vi "FeedbackDecode_20200902.vi"() -> ()   [LabVIEW 2016] (continued)
                n1304 = call "FeedbackDecode_WriteTextEOL.vi"("text"=w1184, "refnum in"=w1190) -> ()  [unwired: 8 in, 2 out]
                n1305 = Initialize Array(0.0 ("element"), 2 ("dimension size"), 12 ("dimension size")) -> (w1179:dbl[][])
                n1306 = Bundle By Name(cluster=w1191, "EventStr"=w1184, "TrialCnt"=w1179) -> (w1183:T5)
                n1307 = local read "LoopCnt"() -> (w1193:u64)
                n1308 = local write "ResetCorr"(TRUE ("ResetCorr")) -> ()
                n1309 = call "FeedbackDecode_MLComCtrl.vi"("DecodeClustIn"=w1183, "Mode"=T19."SendEvent") -> ("DecodeClustOut"=w1178:T5)  [unwired: 6 in, 3 out]
                n1310 = local write "BaseCnt1"(w1193) -> ()
                n1311 = local write "DecodeClust"(w1178) -> ()
              }
            }
          }
          event Value Change {
            n1312 = event-data() -> ("CtlRef"=w1205:refnum<vi>)  [unwired: 1 in, 5 out]
            n1313 = property class="Ctl"(reference=w1205) -> ("Label.Text"=w1204:string)  [unwired: 1 in, 2 out]
            n1314 = case shown="\"ResetTrial\"" w1204 {
              frame "", Default {
              }
              frame "ResetTrial" {
                n1315 = local read "State"() -> (w1207:T16)
                n1316 = case shown="\"Acquire Start\", Default" w1207 {
                  frame "Initialize" {
                    n1317 = local read "DecodeClust"() -> (w1210:T5)
                    n1318 = Bundle By Name(cluster=w1210, "CtrlButtons.ResetTrial"=FALSE) -> (w1209:T5)
                    n1319 = local write "DecodeClust"(w1209) -> ()
                  }
                  frame "Acquire Start", Default {
                    n1320 = local read "NIPTime"() -> (w1215:dbl)
                    n1321 = local read "LoopCnt"() -> (w1219:u64)
                    n1322 = call-poly "FeedbackDecode_VariablesToString.vi"("Format"="%0.0f", "ValueIn"=w1215, "FieldName"="NIPTime" ("Key Word")) -> ("StringOut"=w1212:string)  [unwired: 4 in]
                    n1323 = Format Into String(w1219) -> (resulting string=w1211:string)  [unwired: 3 in, 1 out]
                    n1324 = local read "EventParamsFID"() -> (w1223:refnum<file>)
                    n1325 = local read "DecodeClust"() -> (w1224:T5)
                    n1326 = Concatenate Strings("ResetTrial:SS.EventID=" ("string"), w1211) -> (w1218:string)
                    n1327 = Concatenate Strings(w1218, ";", w1212) -> (w1217:string)
                    n1328 = call "FeedbackDecode_WriteTextEOL.vi"("text"=w1217, "refnum in"=w1223) -> ()  [unwired: 8 in, 2 out]
                    n1329 = Bundle By Name(cluster=w1224, "EventStr"=w1217) -> (w1216:T5)
                    n1330 = call "FeedbackDecode_MLComCtrl.vi"("DecodeClustIn"=w1216, "Mode"=T19."SendEvent") -> ()  [unwired: 6 in, 4 out]
                  }
                }
              }
            }
            n1331 = local read "MvntBuilder"() -> (w1196:T6)
            n1332 = Unbundle By Name(w1196) -> ("Mode"=w1203:enum16{"Selected", "Block", "Random"}, "NTrials"=w1200:dbl, "MvntList"=w1199:T24)
            n1333 = property on="MvntList" class="Arr (strict)"() -> ("Index Values"=w1197:u32[])  [unwired: 2 in, 2 out]
            n1334 = Array Size(array=w1199) -> (size(s)=w1198:i32)
            n1335 = Index Array(array=w1197) -> (element=w1201:u32)  [unwired: 1 in]
            n1336 = call "FeedbackDecode_GenRandBlockIdxs2.vi"("Mode"=w1203, "Reset"=TRUE, "NumTrials"=w1200, "NumIdxs"=w1198, "CurrIdx"=w1201) -> ("Perc"=w1195:dbl)  [unwired: 1 out]
            n1337 = Bundle By Name(cluster=w1196, "PercTrials"=w1195) -> (w1194:T6)
            n1338 = local write "MvntBuilder"(w1194) -> ()
          }
          event Value Change {
            n1339 = event-data() -> ("NewVal"=w1225:bool)  [unwired: 1 in, 5 out]
            n1340 = case shown="True" w1225 {
              frame False {
                n1341 = local read "LoopCnt"() -> (w1237:u64)
                n1342 = local read "NIPTime"() -> (w1231:dbl)
                n1343 = Format Into String(w1237) -> (resulting string=w1227:string)  [unwired: 3 in, 1 out]
                n1344 = call-poly "FeedbackDecode_VariablesToString.vi"("Format"="%0.0f", "ValueIn"=w1231, "FieldName"="NIPTime" ("Key Word")) -> ("StringOut"=w1228:string)  [unwired: 4 in]
                n1345 = Concatenate Strings("DisableHideSpheres:SS.EventID=" ("string"), w1227) -> (w1236:string)
                n1346 = local read "EventParamsFID"() -> (w1234:refnum<file>)
                n1347 = local read "DecodeClust"() -> (w1240:T5)
                n1348 = Concatenate Strings(w1236, ";SS.HideSpheres=0;" ("EventStr"), w1228) -> (w1233:string)
                n1349 = call "FeedbackDecode_WriteTextEOL.vi"("text"=w1233, "refnum in"=w1234) -> ()  [unwired: 8 in, 2 out]
                n1350 = Bundle By Name(cluster=w1240, "EventStr"=w1233) -> (w1232:T5)
                n1351 = call "FeedbackDecode_MLComCtrl.vi"("DecodeClustIn"=w1232, "Mode"=T19."SendEvent") -> ()  [unwired: 6 in, 4 out]
              }
              frame True {
                n1352 = local read "LoopCnt"() -> (w1251:u64)
                n1353 = local read "NIPTime"() -> (w1245:dbl)
                n1354 = Format Into String(w1251) -> (resulting string=w1241:string)  [unwired: 3 in, 1 out]
                n1355 = Concatenate Strings("EnableHideSpheres:SS.EventID=" ("string"), w1241) -> (w1250:string)
                n1356 = call-poly "FeedbackDecode_VariablesToString.vi"("Format"="%0.0f", "ValueIn"=w1245, "FieldName"="NIPTime" ("Key Word")) -> ("StringOut"=w1242:string)  [unwired: 4 in]
                n1357 = local read "EventParamsFID"() -> (w1248:refnum<file>)
                n1358 = local read "DecodeClust"() -> (w1254:T5)
                n1359 = Concatenate Strings(w1250, ";SS.HideSpheres=1;" ("EventStr"), w1242) -> (w1247:string)
                n1360 = call "FeedbackDecode_WriteTextEOL.vi"("text"=w1247, "refnum in"=w1248) -> ()  [unwired: 8 in, 2 out]
                n1361 = Bundle By Name(cluster=w1254, "EventStr"=w1247) -> (w1246:T5)
                n1362 = call "FeedbackDecode_MLComCtrl.vi"("DecodeClustIn"=w1246, "Mode"=T19."SendEvent") -> ()  [unwired: 6 in, 4 out]
              }
            }
          }
          event Value Change {
            n1363 = event-data() -> ("NewVal"=w1256:T44)  [unwired: 1 in, 5 out]
            n1364 = Format Into String(w1256) -> (resulting string=w1255:string)  [unwired: 3 in, 1 out]
            n1365 = local read "LoopCnt"() -> (w1265:u64)
            n1366 = call-poly "FeedbackDecode_VariablesToString.vi"("ValueIn"=w1255, "FieldName"="KalmanType") -> ("StringOut"=w1272:string)  [unwired: 5 in]
            n1367 = local read "NIPTime"() -> (w1261:dbl)
            n1368 = Format Into String(w1265) -> (resulting string=w1257:string)  [unwired: 3 in, 1 out]
            n1369 = local read "EventParamsFID"() -> (w1269:refnum<file>)
            n1370 = local read "DecodeClust"() -> (w1270:T5)
            n1371 = Concatenate Strings("ChangeKalmanType:SS.EventID=" ("string"), w1257) -> (w1264:string)
            n1372 = call-poly "FeedbackDecode_VariablesToString.vi"("Format"="%0.0f", "ValueIn"=w1261, "FieldName"="NIPTime" ("Key Word")) -> ("StringOut"=w1258:string)  [unwired: 4 in]
            n1373 = Concatenate Strings(w1264, ";", w1272, w1258) -> (w1263:string)
            n1374 = call "FeedbackDecode_WriteTextEOL.vi"("text"=w1263, "refnum in"=w1269) -> ()  [unwired: 8 in, 2 out]
            n1375 = Bundle By Name(cluster=w1270, "EventStr"=w1263) -> (w1262:T5)
            n1376 = call "FeedbackDecode_MLComCtrl.vi"("DecodeClustIn"=w1262, "Mode"=T19."SendEvent") -> ()  [unwired: 6 in, 4 out]
          }
          event Value Change {
            n1377 = event-data() -> ()  [unwired: 1 in, 6 out]
            n1378 = call "Load NN"("prompt"="select a .mat file that contains the trained NN") -> ("selected path"=w1276:path)  [unwired: 11 in, 3 out]
            n1379 = Path To String(path=w1276) -> (string=w1275:string)
            n1380 = local read "LoopCnt"() -> (w1285:u64)
            n1381 = call-poly "FeedbackDecode_VariablesToString.vi"("ValueIn"=w1275, "FieldName"="NN.path") -> ("StringOut"=w1292:string)  [unwired: 5 in]
            n1382 = local read "NIPTime"() -> (w1281:dbl)
            n1383 = Format Into String(w1285) -> (resulting string=w1277:string)  [unwired: 3 in, 1 out]
            n1384 = local read "EventParamsFID"() -> (w1289:refnum<file>)
            n1385 = Concatenate Strings("LoadNN:SS.EventID=" ("string"), w1277) -> (w1284:string)
            n1386 = call-poly "FeedbackDecode_VariablesToString.vi"("Format"="%0.0f", "ValueIn"=w1281, "FieldName"="NIPTime" ("Key Word")) -> ("StringOut"=w1278:string)  [unwired: 4 in]
            n1387 = Concatenate Strings(w1284, ";", w1292, w1278) -> (w1283:string)
            n1388 = local read "DecodeClust"() -> (w1290:T5)
            n1389 = call "FeedbackDecode_WriteTextEOL.vi"("text"=w1283, "refnum in"=w1289) -> ()  [unwired: 8 in, 2 out]
            n1390 = Bundle By Name(cluster=w1290, "EventStr"=w1283) -> (w1282:T5)
            n1391 = call "FeedbackDecode_MLComCtrl.vi"("DecodeClustIn"=w1282, "Mode"=T19."SendEvent") -> ()  [unwired: 6 in, 4 out]
          }
          event "CalibrateTASKA": Value Change {
            n1392 = event-data() -> ()  [unwired: 1 in, 6 out]
            n1393 = local read "LoopCnt"() -> (w1302:u64)
            n1394 = local read "NIPTime"() -> (w1298:dbl)
            n1395 = Format Into String(w1302) -> (resulting string=w1294:string)  [unwired: 3 in, 1 out]
            n1396 = local read "EventParamsFID"() -> (w1306:refnum<file>)
            n1397 = Concatenate Strings("CalibrateTASKA:SS.EventID=" ("string"), w1294) -> (w1301:string)
            n1398 = call-poly "FeedbackDecode_VariablesToString.vi"("Format"="%0.0f", "ValueIn"=w1298, "FieldName"="NIPTime" ("Key Word")) -> ("StringOut"=w1295:string)  [unwired: 4 in]
            n1399 = Concatenate Strings(w1301, ";", w1295) -> (w1300:string)
            n1400 = local read "DecodeClust"() -> (w1307:T5)
            n1401 = call "FeedbackDecode_WriteTextEOL.vi"("text"=w1300, "refnum in"=w1306) -> ()  [unwired: 8 in, 2 out]
            n1402 = Bundle By Name(cluster=w1307, "EventStr"=w1300) -> (w1299:T5)
            n1403 = call "FeedbackDecode_MLComCtrl.vi"("DecodeClustIn"=w1299, "Mode"=T19."SendEvent") -> ()  [unwired: 6 in, 4 out]
          }
          event "Reset Calibration": Value Change {
            n1404 = event-data() -> ()  [unwired: 1 in, 6 out]
            n1405 = local read "LoopCnt"() -> (w1317:u64)
            n1406 = local read "NIPTime"() -> (w1313:dbl)
            n1407 = Format Into String(w1317) -> (resulting string=w1309:string)  [unwired: 3 in, 1 out]
            n1408 = local read "EventParamsFID"() -> (w1321:refnum<file>)
            n1409 = Concatenate Strings("CalibrateTASKAreset:SS.EventID=" ("string"), w1309) -> (w1316:string)
            n1410 = call-poly "FeedbackDecode_VariablesToString.vi"("Format"="%0.0f", "ValueIn"=w1313, "FieldName"="NIPTime" ("Key Word")) -> ("StringOut"=w1310:string)  [unwired: 4 in]
            n1411 = Concatenate Strings(w1316, ";", w1310) -> (w1315:string)
            n1412 = local read "DecodeClust"() -> (w1322:T5)
            n1413 = call "FeedbackDecode_WriteTextEOL.vi"("text"=w1315, "refnum in"=w1321) -> ()  [unwired: 8 in, 2 out]
            n1414 = Bundle By Name(cluster=w1322, "EventStr"=w1315) -> (w1314:T5)
            n1415 = call "FeedbackDecode_MLComCtrl.vi"("DecodeClustIn"=w1314, "Mode"=T19."SendEvent") -> ()  [unwired: 6 in, 4 out]
          }
          event "LoadCyberGlove": Value Change {
            n1416 = event-data() -> ()  [unwired: 1 in, 6 out]
            n1417 = call "Load NN2"("prompt"="select a .mat file that contains the cyberglove calibration") -> ("selected path"=w1326:path)  [unwired: 11 in, 3 out]
            n1418 = Path To String(path=w1326) -> (string=w1325:string)
            n1419 = local read "LoopCnt"() -> (w1335:u64)
            n1420 = call-poly "FeedbackDecode_VariablesToString.vi"("ValueIn"=w1325, "FieldName"="CyberGlove.Calibration") -> ("StringOut"=w1342:string)  [unwired: 5 in]
            n1421 = local read "NIPTime"() -> (w1331:dbl)
            n1422 = Format Into String(w1335) -> (resulting string=w1327:string)  [unwired: 3 in, 1 out]
            n1423 = local read "EventParamsFID"() -> (w1339:refnum<file>)
            n1424 = local read "DecodeClust"() -> (w1340:T5)
            n1425 = Concatenate Strings("LoadCyberGlove:SS.EventID=" ("string"), w1327) -> (w1334:string)
            n1426 = call-poly "FeedbackDecode_VariablesToString.vi"("Format"="%0.0f", "ValueIn"=w1331, "FieldName"="NIPTime" ("Key Word")) -> ("StringOut"=w1328:string)  [unwired: 4 in]
            n1427 = Concatenate Strings(w1334, ";", w1342, w1328) -> (w1333:string)
            n1428 = call "FeedbackDecode_WriteTextEOL.vi"("text"=w1333, "refnum in"=w1339) -> ()  [unwired: 8 in, 2 out]
            n1429 = Bundle By Name(cluster=w1340, "EventStr"=w1333) -> (w1332:T5)
            n1430 = call "FeedbackDecode_MLComCtrl.vi"("DecodeClustIn"=w1332, "Mode"=T19."SendEvent") -> ()  [unwired: 6 in, 4 out]
          }
          event "Stim Thresholds": Value Change {
            # "convert from Newtons to 0 to 1 sensor value"
            n1431 = event-data() -> ("NewVal"=w1346:dbl[])  [unwired: 1 in, 5 out]
            n1432 = Divide(x=w1346, y=25.5) -> (x/y=w1347:dbl[])
            n1433 = local read "LoopCnt"() -> (w1356:u64)
            n1434 = call-poly "FeedbackDecode_VariablesToString.vi"("Format"="%0.6f", "ValueIn"=w1347, "FieldName"="DEKA.SensorThresholds") -> ("StringOut"=w1363:string)  [unwired: 4 in]
            n1435 = local read "NIPTime"() -> (w1352:dbl)
            n1436 = Format Into String(w1356) -> (resulting string=w1348:string)  [unwired: 3 in, 1 out]
            n1437 = local read "EventParamsFID"() -> (w1360:refnum<file>)
            n1438 = local read "DecodeClust"() -> (w1361:T5)
            n1439 = Concatenate Strings("UpdateSensorThresholds:SS.EventID=" ("string"), w1348) -> (w1355:string)
            n1440 = call-poly "FeedbackDecode_VariablesToString.vi"("Format"="%0.0f", "ValueIn"=w1352, "FieldName"="NIPTime" ("Key Word")) -> ("StringOut"=w1349:string)  [unwired: 4 in]
            n1441 = Concatenate Strings(w1355, ";", w1363, w1349) -> (w1354:string)
            n1442 = call "FeedbackDecode_WriteTextEOL.vi"("text"=w1354, "refnum in"=w1360) -> ()  [unwired: 8 in, 2 out]
            n1443 = Bundle By Name(cluster=w1361, "EventStr"=w1354) -> (w1353:T5)
            n1444 = call "FeedbackDecode_MLComCtrl.vi"("DecodeClustIn"=w1353, "Mode"=T19."SendEvent") -> ()  [unwired: 6 in, 4 out]
          }
          event Value Change {
            n1445 = event-data() -> ("NewVal"=w1371:string)  [unwired: 1 in, 5 out]
            n1446 = local read "LoopCnt"() -> (w1374:u64)
            n1447 = local read "NIPTime"() -> (w1369:dbl)
            n1448 = Format Into String(w1374) -> (resulting string=w1365:string)  [unwired: 3 in, 1 out]
            n1449 = local read "DecodeClust"() -> (w1379:T5)
            n1450 = Concatenate Strings("SS.LinkedDOF=" ("FieldName"), w1371, ";" ("string")) -> (w1382:string)
            n1451 = local read "EventParamsFID"() -> (w1378:refnum<file>)
            n1452 = Concatenate Strings("LinkDOF:SS.EventID=" ("string"), w1365) -> (w1373:string)
            n1453 = call-poly "FeedbackDecode_VariablesToString.vi"("Format"="%0.0f", "ValueIn"=w1369, "FieldName"="NIPTime" ("Key Word")) -> ("StringOut"=w1366:string)  [unwired: 4 in]
            n1454 = Concatenate Strings(w1373, ";", w1382, w1366) -> (w1372:string)
            n1455 = call "FeedbackDecode_WriteTextEOL.vi"("text"=w1372, "refnum in"=w1378) -> ()  [unwired: 8 in, 2 out]
            n1456 = Bundle By Name(cluster=w1379, "EventStr"=w1372) -> (w1370:T5)
            n1457 = call "FeedbackDecode_MLComCtrl.vi"("DecodeClustIn"=w1370, "Mode"=T19."SendEvent") -> ()  [unwired: 6 in, 4 out]
          }
          event Value Change {
            n1458 = event-data() -> ("NewVal"=w1390:enum16{"Standard", "Stepwise", "Gram"})  [unwired: 1 in, 5 out]
            n1459 = local read "LoopCnt"() -> (w1393:u64)
            n1460 = call-poly "FeedbackDecode_VariablesToString.vi"("Format"="%0.0f", "ValueIn"=w1390, "FieldName"="AutoPopType") -> ("StringOut"=w1401:string)  [unwired: 4 in]
            n1461 = local read "NIPTime"() -> (w1388:dbl)
            n1462 = Format Into String(w1393) -> (resulting string=w1384:string)  [unwired: 3 in, 1 out]
            n1463 = local read "EventParamsFID"() -> (w1397:refnum<file>)
            n1464 = local read "DecodeClust"() -> (w1398:T5)
            n1465 = Concatenate Strings("ChangeAutoPopType:SS.EventID=" ("string"), w1384) -> (w1392:string)
            n1466 = call-poly "FeedbackDecode_VariablesToString.vi"("Format"="%0.0f", "ValueIn"=w1388, "FieldName"="NIPTime" ("Key Word")) -> ("StringOut"=w1385:string)  [unwired: 4 in]
            n1467 = Concatenate Strings(w1392, ";", w1401, w1385) -> (w1391:string)
            n1468 = call "FeedbackDecode_WriteTextEOL.vi"("text"=w1391, "refnum in"=w1397) -> ()  [unwired: 8 in, 2 out]
            n1469 = Bundle By Name(cluster=w1398, "EventStr"=w1391) -> (w1389:T5)
            n1470 = call "FeedbackDecode_MLComCtrl.vi"("DecodeClustIn"=w1389, "Mode"=T19."SendEvent") -> ()  [unwired: 6 in, 4 out]
          }
          event Value Change {
            n1471 = event-data() -> ("NewVal"=w1404:enum16{"Standard", "NN"})  [unwired: 1 in, 5 out]
            n1472 = Format Into String(w1404) -> (resulting string=w1403:string)  [unwired: 3 in, 1 out]
            n1473 = local read "LoopCnt"() -> (w1413:u64)
            n1474 = call-poly "FeedbackDecode_VariablesToString.vi"("ValueIn"=w1403, "FieldName"="CARType") -> ("StringOut"=w1420:string)  [unwired: 5 in]
            n1475 = local read "NIPTime"() -> (w1409:dbl)
            n1476 = Format Into String(w1413) -> (resulting string=w1405:string)  [unwired: 3 in, 1 out]
            n1477 = local read "EventParamsFID"() -> (w1417:refnum<file>)
            n1478 = Concatenate Strings("ChangeCARType:SS.EventID=" ("string"), w1405) -> (w1412:string)
            n1479 = local read "DecodeClust"() -> (w1418:T5)
            n1480 = call-poly "FeedbackDecode_VariablesToString.vi"("Format"="%0.0f", "ValueIn"=w1409, "FieldName"="NIPTime" ("Key Word")) -> ("StringOut"=w1406:string)  [unwired: 4 in]
            n1481 = Concatenate Strings(w1412, ";", w1420, w1406) -> (w1411:string)
            n1482 = call "FeedbackDecode_WriteTextEOL.vi"("text"=w1411, "refnum in"=w1417) -> ()  [unwired: 8 in, 2 out]
            n1483 = Bundle By Name(cluster=w1418, "EventStr"=w1411) -> (w1410:T5)
            n1484 = call "FeedbackDecode_MLComCtrl.vi"("DecodeClustIn"=w1410, "Mode"=T19."SendEvent") -> ()  [unwired: 6 in, 4 out]
          }
          event Value Change {
            n1485 = event-data() -> ("NewVal"=w1424:bool)  [unwired: 1 in, 5 out]
            n1486 = Boolean To (0,1)(Boolean=w1424) -> (0, 1=w1423:i16)
            n1487 = local read "LoopCnt"() -> (w1433:u64)
            n1488 = call-poly "FeedbackDecode_VariablesToString.vi"("Format"="%0.0f", "ValueIn"=w1423, "FieldName"="LimitExt") -> ("StringOut"=w1440:string)  [unwired: 4 in]
            n1489 = local read "NIPTime"() -> (w1429:dbl)
            n1490 = Format Into String(w1433) -> (resulting string=w1425:string)  [unwired: 3 in, 1 out]
            n1491 = local read "DecodeClust"() -> (w1438:T5)
            n1492 = local read "EventParamsFID"() -> (w1437:refnum<file>)
            n1493 = Concatenate Strings("LimitExt:SS.EventID=" ("string"), w1425) -> (w1432:string)
            n1494 = call-poly "FeedbackDecode_VariablesToString.vi"("Format"="%0.0f", "ValueIn"=w1429, "FieldName"="NIPTime" ("Key Word")) -> ("StringOut"=w1426:string)  [unwired: 4 in]
            n1495 = Concatenate Strings(w1432, ";", w1440, w1426) -> (w1431:string)
            n1496 = call "FeedbackDecode_WriteTextEOL.vi"("text"=w1431, "refnum in"=w1437) -> ()  [unwired: 8 in, 2 out]
            n1497 = Bundle By Name(cluster=w1438, "EventStr"=w1431) -> (w1430:T5)
            n1498 = call "FeedbackDecode_MLComCtrl.vi"("DecodeClustIn"=w1430, "Mode"=T19."SendEvent") -> ()  [unwired: 6 in, 4 out]
          }
          event Value Change {
            n1499 = event-data() -> ("NewVal"=w1444:bool)  [unwired: 1 in, 5 out]
            n1500 = Boolean To (0,1)(Boolean=w1444) -> (0, 1=w1443:i16)
            n1501 = local read "LoopCnt"() -> (w1453:u64)
            n1502 = call-poly "FeedbackDecode_VariablesToString.vi"("Format"="%0.0f", "ValueIn"=w1443, "FieldName"="DynFlag") -> ("StringOut"=w1460:string)  [unwired: 4 in]
            n1503 = local read "NIPTime"() -> (w1449:dbl)
            n1504 = Format Into String(w1453) -> (resulting string=w1445:string)  [unwired: 3 in, 1 out]
            n1505 = local read "DecodeClust"() -> (w1458:T5)
            n1506 = local read "EventParamsFID"() -> (w1457:refnum<file>)
            n1507 = Concatenate Strings("DynFlag:SS.EventID=" ("string"), w1445) -> (w1452:string)
            n1508 = call-poly "FeedbackDecode_VariablesToString.vi"("Format"="%0.0f", "ValueIn"=w1449, "FieldName"="NIPTime" ("Key Word")) -> ("StringOut"=w1446:string)  [unwired: 4 in]
            n1509 = Concatenate Strings(w1452, ";", w1460, w1446) -> (w1451:string)
            n1510 = call "FeedbackDecode_WriteTextEOL.vi"("text"=w1451, "refnum in"=w1457) -> ()  [unwired: 8 in, 2 out]
            n1511 = Bundle By Name(cluster=w1458, "EventStr"=w1451) -> (w1450:T5)
            n1512 = call "FeedbackDecode_MLComCtrl.vi"("DecodeClustIn"=w1450, "Mode"=T19."SendEvent") -> ()  [unwired: 6 in, 4 out]
          }
          event Mouse Move {
            n1513 = event-data() -> ("Coords"=w1469:T45)  [unwired: 1 in, 3 out]
            n1514 = local read "HoverPicPos"() -> (w1467:T14)
            n1515 = call "FeedbackDecode_HoverElect.vi"("Border"=2.0, "PicPos"=w1467, "MousePos"=w1469, "Mode"=enum16{"Initialize", "Run"}."Run") -> ("Elect"=w1462:i32)  [unwired: 2 in, 1 out]
            n1516 = local read "DecodeClust"() -> (w1464:T5)
            n1517 = Bundle By Name(cluster=w1464, "HoverElect"=w1462) -> (w1463:T5)
            n1518 = local write "DecodeClust"(w1463) -> ()
          }
          event Value Change {
            # "Also updated CtrlMode and CtrlSpd"
            n1519 = event-data() -> ()  [unwired: 1 in, 6 out]
            n1520 = local read "DecodeClust"() -> (w1475:T5)
            n1521 = Unbundle By Name(w1475) -> ("KMvntClust"=w1476:T46)
            n1522 = call "FeedbackDecode_KalmanMvnts2Str.vi"("KMvntClust"=w1476) -> ("KMvntStr"=w1472:string)
            n1523 = Concatenate Strings("UpdateKGainThresh:" ("string"), w1472) -> (w1471:string)
            n1524 = Bundle By Name(cluster=w1475, "EventStr"=w1471) -> (w1470:T5)
            n1525 = call "FeedbackDecode_MLComCtrl.vi"("DecodeClustIn"=w1470, "Mode"=T19."SendEvent") -> ()  [unwired: 6 in, 4 out]
          }
          event Value Change {
            n1526 = event-data() -> ("NewVal"=w1479:bool)  [unwired: 1 in, 5 out]
            n1527 = case shown="True" w1479 {
              frame False {
              }
              frame True {
                n1528 = local read "DecodeClust"() -> (w1503:T5)
                n1529 = Unbundle By Name(w1503) -> ("ThreshMode"=w1481:T47, "ThreshVal"=w1498:dbl)
                n1530 = Format Into String(w1481) -> (resulting string=w1480:string)  [unwired: 3 in, 1 out]
                n1531 = local read "LoopCnt"() -> (w1492:u64)
                n1532 = call-poly "FeedbackDecode_VariablesToString.vi"("ValueIn"=w1480, "FieldName"="ThreshMode") -> ("StringOut"=w1500:string)  [unwired: 5 in]
                n1533 = call-poly "FeedbackDecode_VariablesToString.vi"("ValueIn"=w1498, "FieldName"="ThreshVal") -> ("StringOut"=w1497:string)  [unwired: 5 in]
                n1534 = local read "NIPTime"() -> (w1486:dbl)
                n1535 = Concatenate Strings(w1500, w1497) -> (w1502:string)
                n1536 = Format Into String(w1492) -> (resulting string=w1482:string)  [unwired: 3 in, 1 out]
                n1537 = local read "EventParamsFID"() -> (w1496:refnum<file>)
                n1538 = call-poly "FeedbackDecode_VariablesToString.vi"("Format"="%0.0f", "ValueIn"=w1486, "FieldName"="NIPTime" ("Key Word")) -> ("StringOut"=w1483:string)  [unwired: 4 in]
                n1539 = Concatenate Strings("UpdateThresh:SS.EventID=" ("string"), w1482) -> (w1491:string)
                n1540 = Concatenate Strings(w1491, ";", w1502, w1483) -> (w1490:string)
                n1541 = call "FeedbackDecode_WriteTextEOL.vi"("text"=w1490, "refnum in"=w1496) -> ()  [unwired: 8 in, 2 out]
                n1542 = Bundle By Name(cluster=w1503, "EventStr"=w1490, "ApplyThresh"=FALSE) -> (w1489:T5)
                n1543 = call "FeedbackDecode_MLComCtrl.vi"("DecodeClustIn"=w1489, "Mode"=T19."SendEvent") -> ("DecodeClustOut"=w1487:T5)  [unwired: 6 in, 3 out]
                n1544 = local write "DecodeClust"(w1487) -> ()
              }
            }
          }
          event Value Change {
            n1545 = event-data() -> ("NewVal"=w1508:dbl)  [unwired: 1 in, 5 out]
            n1546 = Divide(x=w1508, y=0.033) -> (x/y=w1504:dbl)
            n1547 = Multiply(x=2.0, y=w1504) -> (x*y=w1506:dbl)
            n1548 = property on="SelData" class="WFGraph (strict)"("XScale.Maximum"=w1506) -> ()  [unwired: 2 in, 2 out]
            n1549 = property on="SelRate" class="WFGraph (strict)"("XScale.Maximum"=w1504) -> ()  [unwired: 2 in, 2 out]
            n1550 = property on="SelKin" class="WFGraph (strict)"("XScale.Maximum"=w1504) -> ()  [unwired: 2 in, 2 out]
          }
          event Value Change {
            n1551 = event-data() -> ("NewVal"=w1511:bool)  [unwired: 1 in, 5 out]
            n1552 = case shown="True" w1511 {
              frame False {
              }
              frame True {
                n1553 = for {
                  N: 2 -> [_]
                  tunnel: [w1517] -> w1512 mode=indexing
                  n1554 = Initialize Array(FALSE, 100 ("dimension size")) -> (w1518:bool[])
                  n1555 = Array To Cluster(array=w1518) -> (cluster=w1517:T48)
                }
                n1556 = local read "DecodeClust"() -> (w1515:T5)
                n1557 = Bundle By Name(cluster=w1515, "ClearUEA"=FALSE ("CtrlButtons.ResetTrial"), "KUEAArray"=w1512) -> (w1514:T5)
                n1558 = local write "DecodeClust"(w1514) -> ()
              }
            }
          }
          event Value Change {
            n1559 = event-data() -> ("NewVal"=w1522:bool)  [unwired: 1 in, 5 out]
            n1560 = case shown="True" w1522 {
              frame False {
              }
              frame True {
                n1561 = for {
                  N: 2 -> [_]
                  tunnel: [w1528] -> w1523 mode=indexing
                  n1562 = Initialize Array(TRUE, 100 ("dimension size")) -> (w1529:bool[])
                  n1563 = Array To Cluster(array=w1529) -> (cluster=w1528:T48)
                }
                n1564 = local read "DecodeClust"() -> (w1526:T5)
                n1565 = Bundle By Name(cluster=w1526, "FillUEA"=FALSE ("CtrlButtons.ResetTrial"), "KUEAArray"=w1523) -> (w1525:T5)
                n1566 = local write "DecodeClust"(w1525) -> ()
              }
            }
          }
          event Value Change {
            n1567 = event-data() -> ("NewVal"=w1533:bool)  [unwired: 1 in, 5 out]
            n1568 = case shown="True" w1533 {
              frame False {
              }
              frame True {
                n1569 = Initialize Array(FALSE, 80 ("dimension size")) -> (w1539:bool[])
                n1570 = Array To Cluster(array=w1539) -> (cluster=w1535:T49)
                n1571 = local read "DecodeClust"() -> (w1538:T5)
                n1572 = Bundle By Name(cluster=w1538, "ClearEMG"=FALSE ("CtrlButtons.ResetTrial"), "KEMGClust"=w1535, "KEMGExtra"=dbl[] []) -> (w1537:T5)
                n1573 = local write "DecodeClust"(w1537) -> ()
              }
            }
          }
          event Value Change {
            n1574 = event-data() -> ("NewVal"=w1543:bool)  [unwired: 1 in, 5 out]
            n1575 = case shown="True" w1543 {
              frame False {
              }
              frame True {
                n1576 = Initialize Array(TRUE, 80 ("dimension size")) -> (w1548:bool[])
                n1577 = Array To Cluster(array=w1548) -> (cluster=w1544:T49)
                n1578 = local read "DecodeClust"() -> (w1545:T5)
                n1579 = Bundle By Name(cluster=w1545, "FillEMG"=FALSE ("CtrlButtons.ResetTrial"), "KEMGClust"=w1544) -> (w1546:T5)
                n1580 = local write "DecodeClust"(w1546) -> ()
              }
            }
          }
          event Value Change {
            n1581 = event-data() -> ()  [unwired: 1 in, 6 out]
            n1582 = local read "DecodeClust"() -> (w1566:T5)
            n1583 = Unbundle By Name(w1566) -> ("GainFill"=w1565:dbl, "ThreshFill"=w1564:dbl, "ModeFill"=w1555:T50, "SpdFill"=w1552:dbl)
            n1584 = Initialize Array(w1565, 12 ("dimension size"), 2 ("dimension size")) -> (w1570:dbl[][])
            n1585 = Initialize Array(w1564, 12 ("dimension size"), 2 ("dimension size")) -> (w1567:dbl[][])
            n1586 = Initialize Array(w1555, 12 ("dimension size")) -> (w1554:T43)
            n1587 = Initialize Array(w1552, 12 ("dimension size")) -> (w1551:dbl[])
            n1588 = Bundle By Name(cluster=w1566, "KMvntClust.KGain"=w1570, "KMvntClust.KThresh"=w1567, "KMvntClust.CtrlMode"=w1554, "KMvntClust.CtrlSpd"=w1551, "FillMvnts"=FALSE ("ClearKalman")) -> (w1557:T5)
            n1589 = Unbundle By Name(w1557) -> ("KMvntClust"=w1563:T46)
            n1590 = local write "DecodeClust"(w1557) -> ()
            n1591 = call "FeedbackDecode_KalmanMvnts2Str.vi"("KMvntClust"=w1563) -> ("KMvntStr"=w1560:string)
            n1592 = Concatenate Strings("UpdateKGainThresh:" ("string"), w1560) -> (w1559:string)
            n1593 = Bundle By Name(cluster=w1557, "EventStr"=w1559) -> (w1558:T5)
            n1594 = call "FeedbackDecode_MLComCtrl.vi"("DecodeClustIn"=w1558, "Mode"=T19."SendEvent") -> ()  [unwired: 6 in, 4 out]
          }
          event Value Change {
            n1595 = event-data() -> ("NewVal"=w1575:bool)  [unwired: 1 in, 5 out]
            n1596 = case shown="True" w1575 {
              frame False {
              }
              frame True {
                n1597 = Initialize Array(0.0 ("element"), 2 ("dimension size"), 12 ("dimension size")) -> (w1577:dbl[][])
                n1598 = local read "DecodeClust"() -> (w1580:T5)
                n1599 = Bundle By Name(cluster=w1580, "ClearTrials"=FALSE ("CtrlButtons.ResetTrial"), "TrialCnt"=w1577) -> (w1579:T5)
                n1600 = local write "DecodeClust"(w1579) -> ()
              }
            }
          }
          event Value Change {
            n1601 = event-data() -> ("NewVal"=w1590:dbl)  [unwired: 1 in, 5 out]
            n1602 = local read "LoopCnt"() -> (w1593:u64)
            n1603 = local read "NIPTime"() -> (w1588:dbl)
            n1604 = call-poly "FeedbackDecode_VariablesToString.vi"("ValueIn"=w1590, "FieldName"="Lag") -> ("StringOut"=w1600:string)  [unwired: 5 in]
            n1605 = local read "DecodeClust"() -> (w1598:T5)
            n1606 = Format Into String(w1593) -> (resulting string=w1584:string)  [unwired: 3 in, 1 out]
            n1607 = local read "EventParamsFID"() -> (w1597:refnum<file>)
            n1608 = call-poly "FeedbackDecode_VariablesToString.vi"("Format"="%0.0f", "ValueIn"=w1588, "FieldName"="NIPTime" ("Key Word")) -> ("StringOut"=w1585:string)  [unwired: 4 in]
            n1609 = Concatenate Strings("ChangeLag:SS.EventID=" ("string"), w1584) -> (w1592:string)
            n1610 = Concatenate Strings(w1592, ";", w1600, w1585) -> (w1591:string)
            n1611 = call "FeedbackDecode_WriteTextEOL.vi"("text"=w1591, "refnum in"=w1597) -> ()  [unwired: 8 in, 2 out]
            n1612 = Bundle By Name(cluster=w1598, "EventStr"=w1591) -> (w1589:T5)
            n1613 = call "FeedbackDecode_MLComCtrl.vi"("DecodeClustIn"=w1589, "Mode"=T19."SendEvent") -> ()  [unwired: 6 in, 4 out]
          }
          event Value Change {
            n1614 = event-data() -> ("NewVal"=w1608:dbl)  [unwired: 1 in, 5 out]
            n1615 = local read "LoopCnt"() -> (w1611:u64)
            n1616 = local read "NIPTime"() -> (w1606:dbl)
            n1617 = call-poly "FeedbackDecode_VariablesToString.vi"("ValueIn"=w1608, "FieldName"="KernelWidth") -> ("StringOut"=w1618:string)  [unwired: 5 in]
            n1618 = local read "DecodeClust"() -> (w1616:T5)
            n1619 = Format Into String(w1611) -> (resulting string=w1602:string)  [unwired: 3 in, 1 out]
            n1620 = local read "EventParamsFID"() -> (w1615:refnum<file>)
            n1621 = call-poly "FeedbackDecode_VariablesToString.vi"("Format"="%0.0f", "ValueIn"=w1606, "FieldName"="NIPTime" ("Key Word")) -> ("StringOut"=w1603:string)  [unwired: 4 in]
            n1622 = Concatenate Strings("ChangeKernel:SS.EventID=" ("string"), w1602) -> (w1610:string)
            n1623 = Concatenate Strings(w1610, ";", w1618, w1603) -> (w1609:string)
            n1624 = call "FeedbackDecode_WriteTextEOL.vi"("text"=w1609, "refnum in"=w1615) -> ()  [unwired: 8 in, 2 out]
            n1625 = Bundle By Name(cluster=w1616, "EventStr"=w1609) -> (w1607:T5)
            n1626 = call "FeedbackDecode_MLComCtrl.vi"("DecodeClustIn"=w1607, "Mode"=T19."SendEvent") -> ()  [unwired: 6 in, 4 out]
          }
          event Value Change {
            n1627 = event-data() -> ("NewVal"=w1626:dbl)  [unwired: 1 in, 5 out]
            n1628 = local read "LoopCnt"() -> (w1629:u64)
            n1629 = local read "NIPTime"() -> (w1624:dbl)
            n1630 = call-poly "FeedbackDecode_VariablesToString.vi"("ValueIn"=w1626, "FieldName"="TargRad") -> ("StringOut"=w1636:string)  [unwired: 5 in]
            n1631 = local read "DecodeClust"() -> (w1634:T5)
            n1632 = Format Into String(w1629) -> (resulting string=w1620:string)  [unwired: 3 in, 1 out]
            n1633 = local read "EventParamsFID"() -> (w1633:refnum<file>)
            n1634 = call-poly "FeedbackDecode_VariablesToString.vi"("Format"="%0.0f", "ValueIn"=w1624, "FieldName"="NIPTime" ("Key Word")) -> ("StringOut"=w1621:string)  [unwired: 4 in]
            n1635 = Concatenate Strings("ChangeTargRad:SS.EventID=" ("string"), w1620) -> (w1628:string)
            n1636 = Concatenate Strings(w1628, ";", w1636, w1621) -> (w1627:string)
            n1637 = call "FeedbackDecode_WriteTextEOL.vi"("text"=w1627, "refnum in"=w1633) -> ()  [unwired: 8 in, 2 out]
            n1638 = Bundle By Name(cluster=w1634, "EventStr"=w1627) -> (w1625:T5)
            n1639 = call "FeedbackDecode_MLComCtrl.vi"("DecodeClustIn"=w1625, "Mode"=T19."SendEvent") -> ()  [unwired: 6 in, 4 out]
          }
          event Value Change {
            n1640 = event-data() -> ("NewVal"=w1644:T37)  [unwired: 1 in, 5 out]
            n1641 = local read "LoopCnt"() -> (w1647:u64)
            n1642 = Format Into String(w1644) -> (resulting string=w1655:string)  [unwired: 3 in, 1 out]
            n1643 = local read "NIPTime"() -> (w1642:dbl)
            n1644 = local read "DecodeClust"() -> (w1652:T5)
            n1645 = Format Into String(w1647) -> (resulting string=w1638:string)  [unwired: 3 in, 1 out]
            n1646 = Concatenate Strings("SS.KinSrc='" ("string"), w1655, "';" ("string")) -> (w1656:string)
            n1647 = local read "EventParamsFID"() -> (w1651:refnum<file>)
            n1648 = call-poly "FeedbackDecode_VariablesToString.vi"("Format"="%0.0f", "ValueIn"=w1642, "FieldName"="NIPTime" ("Key Word")) -> ("StringOut"=w1639:string)  [unwired: 4 in]
            n1649 = Concatenate Strings("ChangeKinSrc:SS.EventID=" ("string"), w1638) -> (w1646:string)
            n1650 = Concatenate Strings(w1646, ";", w1656, w1639) -> (w1645:string)
            n1651 = call "FeedbackDecode_WriteTextEOL.vi"("text"=w1645, "refnum in"=w1651) -> ()  [unwired: 8 in, 2 out]
            n1652 = Bundle By Name(cluster=w1652, "EventStr"=w1645) -> (w1643:T5)
            n1653 = call "FeedbackDecode_MLComCtrl.vi"("DecodeClustIn"=w1643, "Mode"=T19."SendEvent") -> ()  [unwired: 6 in, 4 out]
          }
          event Value Change {
            n1654 = event-data() -> ("NewVal"=w1658:T23)  [unwired: 1 in, 5 out]
            n1655 = local read "LoopCnt"() -> (w1667:u64)
            n1656 = Format Into String(w1658) -> (resulting string=w1675:string)  [unwired: 3 in, 1 out]
            n1657 = local read "NIPTime"() -> (w1663:dbl)
            n1658 = local read "DecodeClust"() -> (w1672:T5)
            n1659 = Format Into String(w1667) -> (resulting string=w1659:string)  [unwired: 3 in, 1 out]
            n1660 = Concatenate Strings("SS.TestType='" ("string"), w1675, "';" ("string")) -> (w1676:string)
            n1661 = local read "EventParamsFID"() -> (w1671:refnum<file>)
            n1662 = call-poly "FeedbackDecode_VariablesToString.vi"("Format"="%0.0f", "ValueIn"=w1663, "FieldName"="NIPTime" ("Key Word")) -> ("StringOut"=w1660:string)  [unwired: 4 in]
            n1663 = Concatenate Strings("ChangeTestType:SS.EventID=" ("string"), w1659) -> (w1666:string)
            n1664 = Concatenate Strings(w1666, ";", w1676, w1660) -> (w1665:string)
            n1665 = call "FeedbackDecode_WriteTextEOL.vi"("text"=w1665, "refnum in"=w1671) -> ()  [unwired: 8 in, 2 out]
            n1666 = Bundle By Name(cluster=w1672, "EventStr"=w1665) -> (w1664:T5)
            n1667 = call "FeedbackDecode_MLComCtrl.vi"("DecodeClustIn"=w1664, "Mode"=T19."SendEvent") -> ()  [unwired: 6 in, 4 out]
          }
          event Value Change {
            n1668 = event-data() -> ("NewVal"=w1678:bool)  [unwired: 1 in, 5 out]
            n1669 = case shown="True" w1678 {
              frame False {
              }
              frame True {
                n1670 = local read "LoopCnt"() -> (w1691:u64)
                n1671 = local read "NIPTime"() -> (w1684:dbl)
                n1672 = Format Into String(w1691) -> (resulting string=w1680:string)  [unwired: 3 in, 1 out]
                n1673 = local read "EventParamsFID"() -> (w1695:refnum<file>)
                n1674 = call-poly "FeedbackDecode_VariablesToString.vi"("Format"="%0.0f", "ValueIn"=w1684, "FieldName"="NIPTime" ("Key Word")) -> ("StringOut"=w1681:string)  [unwired: 4 in]
                n1675 = Concatenate Strings("ResetVRE:SS.EventID=" ("string"), w1680) -> (w1690:string)
                n1676 = Concatenate Strings(w1690, ";", w1681) -> (w1689:string)
                n1677 = local read "DecodeClust"() -> (w1696:T5)
                n1678 = call "FeedbackDecode_WriteTextEOL.vi"("text"=w1689, "refnum in"=w1695) -> ()  [unwired: 8 in, 2 out]
                n1679 = Bundle By Name(cluster=w1696, "EventStr"=w1689, "CtrlButtons.ResetVRE"=FALSE ("ResetVRE")) -> (w1688:T5)
                n1680 = property on="StimMode" class="Enum (strict)"("Val(Sgnl)"=enum16{"Off", "Manual", "MSMS", "VRE"}."Off" ("Value (Signaling)")) -> ()  [unwired: 2 in, 2 out]
                n1681 = call "FeedbackDecode_MLComCtrl.vi"("DecodeClustIn"=w1688, "Mode"=T19."SendEvent") -> ("DecodeClustOut"=w1686:T5)  [unwired: 6 in, 3 out]
                n1682 = local write "DecodeClust"(w1686) -> ()
              }
            }
          }
          event Value Change {
            n1683 = event-data() -> ("NewVal"=w1697:bool)  [unwired: 1 in, 5 out]
            n1684 = case shown="True" w1697 {
              frame False {
              }
              frame True {
                n1685 = local read "LoopCnt"() -> (w1710:u64)
                n1686 = local read "NIPTime"() -> (w1703:dbl)
                n1687 = Format Into String(w1710) -> (resulting string=w1699:string)  [unwired: 3 in, 1 out]
                n1688 = local read "EventParamsFID"() -> (w1714:refnum<file>)
                n1689 = Concatenate Strings("StopVRE:SS.EventID=" ("string"), w1699) -> (w1709:string)
                n1690 = call-poly "FeedbackDecode_VariablesToString.vi"("Format"="%0.0f", "ValueIn"=w1703, "FieldName"="NIPTime" ("Key Word")) -> ("StringOut"=w1700:string)  [unwired: 4 in]
                n1691 = Concatenate Strings(w1709, ";", w1700) -> (w1708:string)
                n1692 = local read "DecodeClust"() -> (w1715:T5)
                n1693 = call "FeedbackDecode_WriteTextEOL.vi"("text"=w1708, "refnum in"=w1714) -> ()  [unwired: 8 in, 2 out]
                n1694 = Bundle By Name(cluster=w1715, "EventStr"=w1708, "CtrlButtons.StopVRE"=FALSE ("ResetVRE")) -> (w1707:T5)
                n1695 = property on="StimMode" class="Enum (strict)"("Val(Sgnl)"=enum16{"Off", "Manual", "MSMS", "VRE"}."Off" ("Value (Signaling)")) -> ()  [unwired: 2 in, 2 out]
                n1696 = call "FeedbackDecode_MLComCtrl.vi"("DecodeClustIn"=w1707, "Mode"=T19."SendEvent") -> ("DecodeClustOut"=w1705:T5)  [unwired: 6 in, 3 out]
                n1697 = local write "DecodeClust"(w1705) -> ()
              }
            }
          }
          event Value Change {
            n1698 = event-data() -> ("NewVal"=w1716:bool)  [unwired: 1 in, 5 out]
            n1699 = case shown="True" w1716 {
              frame False {
              }
              frame True {
                n1700 = local read "LoopCnt"() -> (w1728:u64)
                n1701 = local read "NIPTime"() -> (w1722:dbl)
                n1702 = Format Into String(w1728) -> (resulting string=w1718:string)  [unwired: 3 in, 1 out]
                n1703 = local read "EventParamsFID"() -> (w1732:refnum<file>)
                n1704 = Concatenate Strings("ConARD:SS.EventID=" ("string"), w1718) -> (w1727:string)
                n1705 = call-poly "FeedbackDecode_VariablesToString.vi"("Format"="%0.0f", "ValueIn"=w1722, "FieldName"="NIPTime" ("Key Word")) -> ("StringOut"=w1719:string)  [unwired: 4 in]
                n1706 = Concatenate Strings(w1727, ";", w1719) -> (w1726:string)
                n1707 = local read "DecodeClust"() -> (w1733:T5)
                n1708 = call "FeedbackDecode_WriteTextEOL.vi"("text"=w1726, "refnum in"=w1732) -> ()  [unwired: 8 in, 2 out]
                n1709 = Bundle By Name(cluster=w1733, "EventStr"=w1726, "CtrlButtons.ConARD"=FALSE ("ResetVRE")) -> (w1725:T5)
                n1710 = call "FeedbackDecode_MLComCtrl.vi"("DecodeClustIn"=w1725, "Mode"=T19."SendEvent") -> ("DecodeClustOut"=w1723:T5)  [unwired: 6 in, 3 out]
                n1711 = local write "DecodeClust"(w1723) -> ()
              }
            }
          }
          event Value Change {
            n1712 = event-data() -> ("NewVal"=w1735:bool)  [unwired: 1 in, 4 out]
            n1713 = case shown="True" w1735 {
              frame False {
              }
              frame True {
                n1714 = property on="MvntList" class="Arr (strict)"() -> ("Index Values"=w1739:u32[])  [unwired: 2 in, 2 out]
                n1715 = local read "MvntBuilder"() -> (w1743:T6)
                n1716 = Index Array(array=w1739) -> (element=w1744:u32)  [unwired: 1 in]
                n1717 = local read "DecodeClust"() -> (w1738:T5)
                n1718 = Bundle By Name(cluster=w1738, "CtrlButtons.StartTrials"=FALSE) -> (w1736:T5)
                n1719 = call "FeedbackDecode_SetMvntBuilder.vi"("MvntBuilderIn"=w1743, "MvntIdx"=w1744) -> ("MvntBuilderOut"=w1742:T6)  [unwired: 1 in]
                n1720 = Bundle By Name(cluster=w1742, "Set"=FALSE) -> (w1740:T6)
                n1721 = local write "MvntBuilder"(w1740) -> ()
                n1722 = local write "DecodeClust"(w1736) -> ()
              }
            }
          }
          event Value Change {
            n1723 = event-data() -> ("NewVal"=w1746:bool)  [unwired: 1 in, 4 out]
            n1724 = case shown="True" w1746 {
              frame False {
              }
              frame True {
                n1725 = local read "MvntBuilder"() -> (w1751:T6)
                n1726 = local read "DecodeClust"() -> (w1750:T5)
                n1727 = Bundle By Name(cluster=w1750, "CtrlButtons.StartTrials"=FALSE) -> (w1748:T5)
                n1728 = Bundle By Name(cluster=w1751, "MvntList"=T24 [], "Clear"=FALSE ("Set")) -> (w1752:T6)
                n1729 = local write "MvntBuilder"(w1752) -> ()
                n1730 = local write "DecodeClust"(w1748) -> ()
              }
            }
          }
          event Value Change {
            n1731 = event-data() -> ("NewVal"=w1755:bool)  [unwired: 1 in, 5 out]
            n1732 = case shown="True" w1755 {
              frame False {
              }
              frame True {
                n1733 = flat-sequence {
                  frame #0 {
                    n1734 = local read "MvntBuilder"() -> (w1759:T6)
                    n1735 = local read "DecodeClust"() -> (w1758:T5)
                    n1736 = Bundle By Name(cluster=w1758, "CtrlButtons.StartTrials"=FALSE) -> (w1756:T5)
                    n1737 = Bundle By Name(cluster=w1759, "Load"=FALSE ("Set")) -> (w1760:T6)
                    n1738 = local write "MvntBuilder"(w1760) -> ()
                    n1739 = local write "DecodeClust"(w1756) -> ()
                  }
                  frame #1 {
                    n1740 = local read "MvntBuilder"() -> (w1763:T6)
                    n1741 = call "FeedbackDecode_MvntListIO.vi"("MvntBuilderIn"=w1763, "Mode"=enum16{"Read", "Write"}."Read") -> ("MvntBuilderOut"=w1762:T6)  [unwired: 1 in]
                    n1742 = Unbundle By Name(w1762) -> ("MvntList"=w1765:T24)
                    n1743 = property on="MvntList" class="Arr (strict)"("Val(Sgnl)"=w1765) -> ()  [unwired: 2 in, 2 out]
                  }
                }
              }
            }
          }
          event Value Change {
            n1744 = event-data() -> ("NewVal"=w1766:bool)  [unwired: 1 in, 5 out]
            n1745 = case shown="True" w1766 {
              frame False {
              }
              frame True {
                n1746 = flat-sequence {
                  frame #0 {
                    n1747 = local read "MvntBuilder"() -> (w1771:T6)
                    n1748 = local read "DecodeClust"() -> (w1770:T5)
                    n1749 = Bundle By Name(cluster=w1770, "CtrlButtons.StartTrials"=FALSE) -> (w1768:T5)
                    n1750 = Bundle By Name(cluster=w1771, "Save"=FALSE ("Set")) -> (w1772:T6)
                    n1751 = local write "MvntBuilder"(w1772) -> ()
                    n1752 = local write "DecodeClust"(w1768) -> ()
                  }
                  frame #1 {
                    n1753 = local read "MvntBuilder"() -> (w1774:T6)
                    n1754 = call "FeedbackDecode_MvntListIO.vi"("MvntBuilderIn"=w1774, "Mode"=enum16{"Read", "Write"}."Write") -> ()  [unwired: 1 in, 1 out]
                  }
                }
              }
            }
          }
          event Value Change {
            n1755 = event-data() -> ("OldVal"=w1779:T24, "NewVal"=w1778:T24)  [unwired: 1 in, 4 out]
            n1756 = Array Size(array=w1779) -> (size(s)=w1780:i32)
            n1757 = Array Size(array=w1778) -> (size(s)=w1781:i32)
            n1758 = Not Equal?(x=w1780, y=w1781) -> (x != y?=w1777:bool)
            n1759 = case shown="True" w1777 {
              frame False {
              }
              frame True {
                n1760 = local read "MvntBuilder"() -> (w1784:T6)
                n1761 = local read "DecodeClust"() -> (w1794:T5)
                n1762 = Bundle By Name(cluster=w1794, "CtrlButtons.StartTrials"=FALSE) -> (w1792:T5)
                n1763 = Unbundle By Name(w1784) -> ("Mode"=w1791:enum16{"Selected", "Block", "Random"}, "NTrials"=w1788:dbl, "MvntList"=w1787:T24)
                n1764 = property on="MvntList" class="Arr (strict)"() -> ("Index Values"=w1785:u32[])  [unwired: 2 in, 2 out]
                n1765 = Array Size(array=w1787) -> (size(s)=w1786:i32)
                n1766 = Index Array(array=w1785) -> (element=w1789:u32)  [unwired: 1 in]
                n1767 = local write "DecodeClust"(w1792) -> ()
                n1768 = call "FeedbackDecode_GenRandBlockIdxs2.vi"("Mode"=w1791, "Reset"=TRUE, "NumTrials"=w1788, "NumIdxs"=w1786, "CurrIdx"=w1789) -> ("Perc"=w1783:dbl)  [unwired: 1 out]
                n1769 = Bundle By Name(cluster=w1784, "PercTrials"=w1783) -> (w1782:T6)
                n1770 = local write "MvntBuilder"(w1782) -> ()
              }
            }
          }
          event Value Change {
            n1771 = event-data() -> ("NewVal"=w1795:dbl)  [unwired: 1 in, 5 out]
            n1772 = local read "MSMSSphere"() -> (w1801:dbl[][])
            n1773 = Initialize Array(w1795, 6 ("dimension size")) -> (w1797:dbl[])
            n1774 = property on="TargRad" class="DigNum (strict)"("Val(Sgnl)"=w1795) -> ()  [unwired: 2 in, 2 out]
            n1775 = Replace Array Subset(array=w1801, new element=w1797, index (col)=3 ("disabled index (col)")) -> (w1800:dbl[][])  [unwired: 1 in]
            n1776 = local write "MSMSSphere"(w1800) -> ()
          }
          event User Event {
            n1777 = event-data() -> ("MvntEvnt"=w1803:dbl)  [unwired: 1 in, 4 out]
            n1778 = Build Array(w1803) -> (w1802:dbl[])
            n1779 = property on="MvntList" class="Arr (strict)"("Index Values"=w1802) -> ()  [unwired: 2 in, 2 out]
          }
          event "MedianHM": Mouse Down {
            w1814 = cluster{"X":i32, "Y":i32} {"X"=0, "Y"=0} ("MousePos")
            w1815 = enum16{"Initialize", "Run", "Mouse"}."Mouse" ("Mode")
            n1780 = event-data() -> ("PlatMods"=w1809:T51, "Coords"=w1812:T45)  [unwired: 1 in, 4 out]
            n1781 = Cluster To Array(cluster=w1809) -> (array=w1808:bool[])
            n1782 = Boolean Array To Number(Boolean array=w1808) -> (number=w1807:u32)
            n1783 = local read "DecodeClust"() -> (w1811:T5)
            n1784 = local read "UEAHMIdx"() -> (w1828:i32[])
            n1785 = call "FeedbackDecode_PlotHeatmap.vi"("MousePos"=w1812, "Instance"=0, "Mode"=w1815) -> ("CurrPos"=w1827:i32)  [unwired: 3 in, 1 out]
            n1786 = call "FeedbackDecode_PlotHeatmap.vi"("MousePos"=w1814, "Instance"=1, "Mode"=w1815) -> ()  [unwired: 3 in, 2 out]
            n1787 = call "FeedbackDecode_PlotHeatmap.vi"("MousePos"=w1814, "Instance"=2, "Mode"=w1815) -> ()  [unwired: 3 in, 2 out]
            n1788 = Search 1D Array(1D array=w1828, element=w1827) -> (index of element=w1826:i32)  [unwired: 1 in]
            n1789 = Increment(x=w1826) -> (x+1=w1813:i32)
            n1790 = case shown="4" w1807 {
              tunnel: w1813 -> [_ w1832 w1836]
              tunnel: w1811 -> [w1829 w1831 w1835]
              tunnel: [w1829 w1830 w1834] -> w1810
              frame 0, Default {
              }
              frame 18 {
                # "ctrl"
                n1791 = call "FeedbackDecode_UpdateDecodeClustElect.vi"("DecodeClustIn"=w1831, "KalmanElect"=w1832) -> ("DecodeClustOut"=w1830:T5)  [unwired: 1 in]
              }
              frame 4 {
                # "alt"
                n1792 = Unbundle By Name(w1835) -> ("BadUEAElects"=w1837:dbl[])
                n1793 = Insert Into Array(array=w1837, new element=w1836) -> (w1833:dbl[])  [unwired: 1 in]
                n1794 = Bundle By Name(cluster=w1835, "BadUEAElects"=w1833) -> (w1834:T5)
                n1795 = property on="BadUEAElects" class="Arr (strict)"("Val(Sgnl)"=w1833) -> ()  [unwired: 2 in, 2 out]
              }
            }
            n1796 = local read "LoopCnt"() -> (w1820:u64)
            n1797 = call-poly "FeedbackDecode_VariablesToString.vi"("Format"="%0.0f", "ValueIn"=w1813, "FieldName"="SelElect") -> ("StringOut"=w1822:string)  [unwired: 4 in]
            n1798 = local write "SelElect"(w1813) -> ()
            n1799 = local write "BaseCnt2"(w1820) -> ()
            n1800 = Bundle By Name(cluster=w1810, "ClearWfs"=TRUE, "SelElect"=w1813, "EventStr"=w1822) -> (w1806:T5)
            n1801 = call "FeedbackDecode_MLComCtrl.vi"("DecodeClustIn"=w1806, "Mode"=T19."SendEvent") -> ("DecodeClustOut"=w1805:T5)  [unwired: 6 in, 3 out]
            n1802 = local write "DecodeClust"(w1805) -> ()
          }
          event "UlnarHM": Mouse Down {
            w1849 = cluster{"X":i32, "Y":i32} {"X"=0, "Y"=0} ("MousePos")
            w1850 = enum16{"Initialize", "Run", "Mouse"}."Mouse" ("Mode")
            n1803 = event-data() -> ("PlatMods"=w1845:T51, "Coords"=w1848:T45)  [unwired: 1 in, 4 out]
            n1804 = Cluster To Array(cluster=w1845) -> (array=w1844:bool[])
            n1805 = local read "DecodeClust"() -> (w1843:T5)
            n1806 = Boolean Array To Number(Boolean array=w1844) -> (number=w1842:u32)
            n1807 = local read "UEAHMIdx"() -> (w1862:i32[])
            n1808 = call "FeedbackDecode_PlotHeatmap.vi"("MousePos"=w1848, "Instance"=1, "Mode"=w1850) -> ("CurrPos"=w1861:i32)  [unwired: 3 in, 1 out]
            n1809 = call "FeedbackDecode_PlotHeatmap.vi"("MousePos"=w1849, "Instance"=0, "Mode"=w1850) -> ()  [unwired: 3 in, 2 out]
            n1810 = call "FeedbackDecode_PlotHeatmap.vi"("MousePos"=w1849, "Instance"=2, "Mode"=w1850) -> ()  [unwired: 3 in, 2 out]
            n1811 = Search 1D Array(1D array=w1862, element=w1861) -> (index of element=w1847:i32)  [unwired: 1 in]
            n1812 = Add(x=w1847, y=101) -> (x+y=w1841:i32)
            n1813 = case shown="4" w1842 {
              tunnel: w1841 -> [_ w1866 w1870]
              tunnel: w1843 -> [w1863 w1865 w1869]
              tunnel: [w1863 w1864 w1868] -> w1840
              frame 0, Default {
              }
              frame 18 {
                # "ctrl"
                n1814 = call "FeedbackDecode_UpdateDecodeClustElect.vi"("DecodeClustIn"=w1865, "KalmanElect"=w1866) -> ("DecodeClustOut"=w1864:T5)  [unwired: 1 in]
              }
              frame 4 {
                # "alt"
                n1815 = Unbundle By Name(w1869) -> ("BadUEAElects"=w1871:dbl[])
                n1816 = Insert Into Array(array=w1871, new element=w1870) -> (w1867:dbl[])  [unwired: 1 in]
                n1817 = Bundle By Name(cluster=w1869, "BadUEAElects"=w1867) -> (w1868:T5)
                n1818 = property on="BadUEAElects" class="Arr (strict)"("Val(Sgnl)"=w1867) -> ()  [unwired: 2 in, 2 out]
              }
            }
            n1819 = local read "LoopCnt"() -> (w1855:u64)
            n1820 = call-poly "FeedbackDecode_VariablesToString.vi"("Format"="%0.0f", "ValueIn"=w1841, "FieldName"="SelElect") -> ("StringOut"=w1857:string)  [unwired: 4 in]
            n1821 = local write "SelElect"(w1841) -> ()
            n1822 = local write "BaseCnt2"(w1855) -> ()
            n1823 = Bundle By Name(cluster=w1840, "ClearWfs"=TRUE, "SelElect"=w1841, "EventStr"=w1857) -> (w1839:T5)
            n1824 = call "FeedbackDecode_MLComCtrl.vi"("DecodeClustIn"=w1839, "Mode"=T19."SendEvent") -> ("DecodeClustOut"=w1838:T5)  [unwired: 6 in, 3 out]
            n1825 = local write "DecodeClust"(w1838) -> ()
          }
          event "EMGHM": Mouse Down {
            w1883 = cluster{"X":i32, "Y":i32} {"X"=0, "Y"=0} ("MousePos")
            w1884 = enum16{"Initialize", "Run", "Mouse"}."Mouse" ("Mode")
            n1826 = event-data() -> ("PlatMods"=w1880:T51, "Coords"=w1882:T45)  [unwired: 1 in, 4 out]
            n1827 = local read "DecodeClust"() -> (w1877:T5)
            n1828 = Cluster To Array(cluster=w1880) -> (array=w1879:bool[])
            n1829 = Boolean Array To Number(Boolean array=w1879) -> (number=w1878:u32)
            n1830 = local read "EMGHMIdx"() -> (w1896:i32[])
            n1831 = call "FeedbackDecode_PlotHeatmap.vi"("MousePos"=w1882, "Instance"=2, "Mode"=w1884) -> ("CurrPos"=w1895:i32)  [unwired: 3 in, 1 out]
            n1832 = call "FeedbackDecode_PlotHeatmap.vi"("MousePos"=w1883, "Instance"=0, "Mode"=w1884) -> ()  [unwired: 3 in, 2 out]
            n1833 = call "FeedbackDecode_PlotHeatmap.vi"("MousePos"=w1883, "Instance"=1, "Mode"=w1884) -> ()  [unwired: 3 in, 2 out]
            n1834 = Search 1D Array(1D array=w1896, element=w1895) -> (index of element=w1874:i32)  [unwired: 1 in]
            n1835 = Add(x=w1874, y=201) -> (x+y=w1876:i32)
            n1836 = case shown="4" w1878 {
              tunnel: w1876 -> [_ w1900 _]
              tunnel: w1877 -> [w1897 w1899 w1905]
              tunnel: [w1897 w1898 w1906] -> w1875
              tunnel: w1874 -> [_ _ w1907]
              frame 0, Default {
              }
              frame 18 {
                # "ctrl"
                n1837 = call "FeedbackDecode_UpdateDecodeClustElect.vi"("DecodeClustIn"=w1899, "KalmanElect"=w1900) -> ("DecodeClustOut"=w1898:T5)  [unwired: 1 in]
              }
              frame 4 {
                # "alt"
                n1838 = Quotient & Remainder(x=w1907, y=10.0) -> (x-y*floor(x/y)=w1911:dbl, floor(x/y)=w1913:dbl)
                n1839 = Increment(x=w1911) -> (x+1=w1912:dbl)
                n1840 = Multiply(x=w1913, y=4.0) -> (x*y=w1910:dbl)
                n1841 = Add(x=w1912, y=w1910) -> (x+y=w1901:dbl)
                n1842 = In Range and Coerce(upper limit=32.0, x=w1901, lower limit=1.0) -> (In Range?=w1902:bool)  [unwired: 1 out]
                n1843 = case shown="True" w1902 {
                  tunnel: w1901 -> [_ w1918]
                  tunnel: [w1914 w1917] -> w1906
                  tunnel: w1905 -> [w1914 w1915]
                  frame False {
                  }
                  frame True {
                    n1844 = Unbundle By Name(w1915) -> ("BadEMGChans"=w1919:dbl[])
                    n1845 = Insert Into Array(array=w1919, new element=w1918) -> (w1916:dbl[])  [unwired: 1 in]
                    n1846 = Bundle By Name(cluster=w1915, "BadEMGChans"=w1916) -> (w1917:T5)
                    n1847 = property on="BadEMGChans" class="Arr (strict)"("Val(Sgnl)"=w1916) -> ()  [unwired: 2 in, 2 out]
                  }
                }
              }
            }
            n1848 = call-poly "FeedbackDecode_VariablesToString.vi"("Format"="%0.0f", "ValueIn"=w1876, "FieldName"="SelElect") -> ("StringOut"=w1891:string)  [unwired: 4 in]
            n1849 = local write "SelElect"(w1876) -> ()
